vi "Update Messages MetaData.vi"(7 "Messages MetaData":T1[](array[typedef]), 8 "error in (no error)":errorcluster, 11 "Library":refnum<vi>) -> (0 "error out":errorcluster, 3 "Library":refnum<vi>)   [LabVIEW 2019, in "gRPC Template Creation Utility.lvlib"]
uses:
  gRPC Template Creation Utility.lvlib
  TypeDefs/Message Metadata (Scripting).ctl
  TypeDefs/Message Element Metadata (Scripting).ctl
  TypeDefs/Message Element Type.ctl
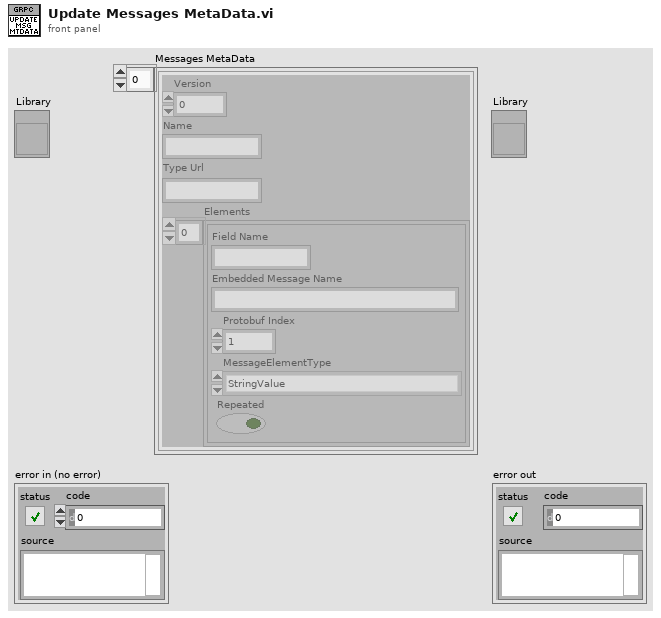
[diagram p1: front panel]
types:
  T1 = typedef "gRPC Template Creation Utility.lvlib/Message Metadata (Scripting).ctl" = cluster{"Version":i32, "Name":string, "Type Url":string, "Elements":T2[]}
  T2 = typedef "gRPC Template Creation Utility.lvlib/Message Element Metadata (Scripting).ctl" = cluster{"Field Name":string, "Embedded Message Name":string, "Protobuf Index":i32, "MessageElementType":T3, "Repeated":bool}
  T3 = typedef "gRPC Template Creation Utility.lvlib/Message Element Type.ctl" = enum32{"Int32Value", "FloatValue", "DoubleValue", "BoolValue", "StringValue", "MessageValue", "Int64Value", "UInt32Value", "UInt64Value", "EnumValue", "Bytes", "Fixed64", "Fixed32", "SFixed64", "SFixed32", "SInt64", "SInt32"}
  T4 = cluster{"Version":i32, "Name":string, "Type Url":string, "Elements":cluster{"Embedded Message Name":string, "Protobuf Index":i32, "MessageElementType":enum32{"Int32Value", "FloatValue", "DoubleValue", "BoolValue", "StringValue", "MessageValue", "Int64Value", "UInt32Value", "UInt64Value", "EnumValue", "Bytes", "Fixed64", "Fixed32", "SFixed64", "SFixed32", "SInt64", "SInt32"}, "Repeated":bool}[]}
  T5 = cluster{"Embedded Message Name":string, "Protobuf Index":i32, "MessageElementType":enum32{"Int32Value", "FloatValue", "DoubleValue", "BoolValue", "StringValue", "MessageValue", "Int64Value", "UInt32Value", "UInt64Value", "EnumValue", "Bytes", "Fixed64", "Fixed32", "SFixed64", "SFixed32", "SInt64", "SInt32"}, "Repeated":bool}
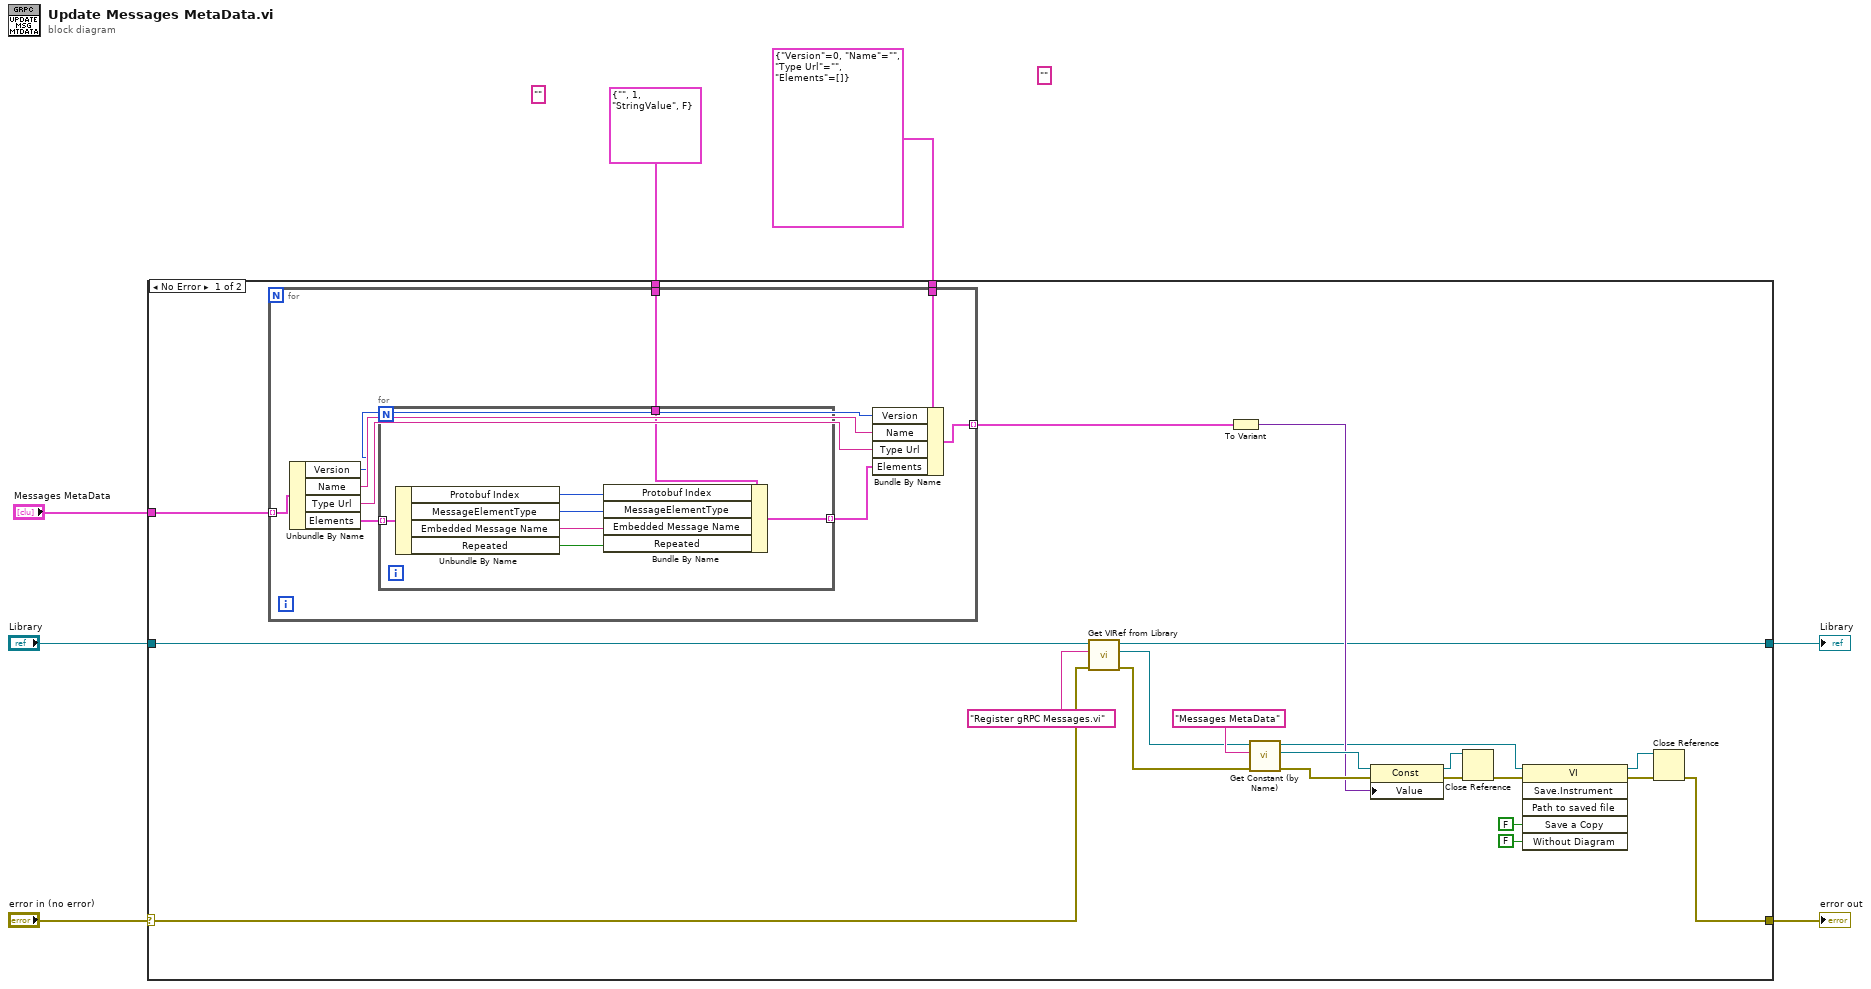
[diagram p0: block diagram]
diagram:
  (unwired) "" ("Field Name")
  (unwired) "" ("Field Name")
  n1 = case shown="No Error" "error in (no error)" {
    selector: "error in (no error)" -> [w18 w47]
    tunnel: [w30 w47] -> w7
    tunnel: [w21 w48] -> w6
    tunnel: "Library" -> [w19 w48]
    tunnel: "Messages MetaData" -> [w17 _]
    tunnel: T5 {"Embedded Message Name"="", "Protobuf Index"=1, "MessageElementType"=enum."StringValue", "Repeated"=FALSE} ("Message Element Metadata") -> [w15 _]
    tunnel: T4 {"Version"=0, "Name"="", "Type Url"="", "Elements"=[]} ("Message Metadata") -> [w14 _]
    frame No Error {
      n2 = for {
        tunnel: w17 -> [w39] mode=indexing
        tunnel: [w37] -> w16 mode=indexing
        tunnel: w15 -> [w32]
        tunnel: w14 -> [w31]
        n3 = Unbundle By Name(w39) -> ("Version"=w33:i32, "Name"=w34:string, "Type Url"=w35:string, "Elements"=w38:T2[])
        n4 = for {
          tunnel: w38 -> [w46] mode=indexing
          tunnel: [w41] -> w36 mode=indexing
          tunnel: w32 -> [w40]
          n5 = Unbundle By Name(w46) -> ("Protobuf Index"=w45:i32, "MessageElementType"=w44:T3, "Embedded Message Name"=w43:string, "Repeated"=w42:bool)
          n6 = Bundle By Name(cluster=w40, "Protobuf Index"=w45, "MessageElementType"=w44, "Embedded Message Name"=w43, "Repeated"=w42) -> (w41:T5)
        }
        n7 = Bundle By Name(cluster=w31, "Version"=w33, "Name"=w34, "Type Url"=w35, "Elements"=w36) -> (w37:T4)
      }
      n8 = call "Get VIRef from Library.vi"("error in (no error)"=w18, "Item Name"="Register gRPC Messages.vi", "Library"=w19) -> ("error out"=w26:errorcluster, "VIref out"=w23:refnum<vi>, "Library"=w21:refnum<vi>)  [unwired: 5 in, 1 out]
      n9 = To Variant(anything=w16) -> (Variant=w22:variant)
      n10 = call "Get Constant (by Name).vi"("error in (no error)"=w26, "Constant Label"="Messages MetaData", "Owner VI in"=w23) -> ("error out"=w27:errorcluster, "Const ref out"=w24:refnum<vi>, "Owner VI out"=w12:refnum<vi>)  [unwired: 5 in, 1 out]
      n11 = property class="Const"(reference=w24, error in=w27, "Value"=w22) -> (reference out=w29:refnum<vi>, error out=w28:errorcluster)
      n12 = Close Reference(reference=w29, error in (no error)=w28) -> (error out=w13:errorcluster)
      n13 = invoke class="VI" method="Save.Instrument"(reference=w12, error in=w13, "Save a Copy"=FALSE, "Without Diagram"=FALSE) -> (reference out=w10:refnum<vi>, error out=w11:errorcluster)  [unwired: 2 in, 4 out]
      n14 = Close Reference(reference=w10, error in (no error)=w11) -> (error out=w30:errorcluster)
    }
    frame Error {
    }
  }
  "error out" <- w7
  "Library" <- w6
